vi "Reconnected.vi"(8 "error in (no error)":errorcluster, 11 "PolledDriver in":refnum<class "PolledDriver.lvclass">) -> (0 "error out":errorcluster, 3 "PolledDriver out":refnum<class "PolledDriver.lvclass">)   [LabVIEW 2013, in "PolledDriver.lvclass"]
doc: "Called when driver has sucesfully reconnected to host"
uses:
  PolledDriver.lvclass
  response.ctl
  driver_status.ctl
  Responder/BaseResponder/BaseResponder.lvclass
  PolledDriver.lvclass/PolledDriver.ctl
  BaseDriver/Read Responder.vi
  BaseDriver/Write Responder.vi
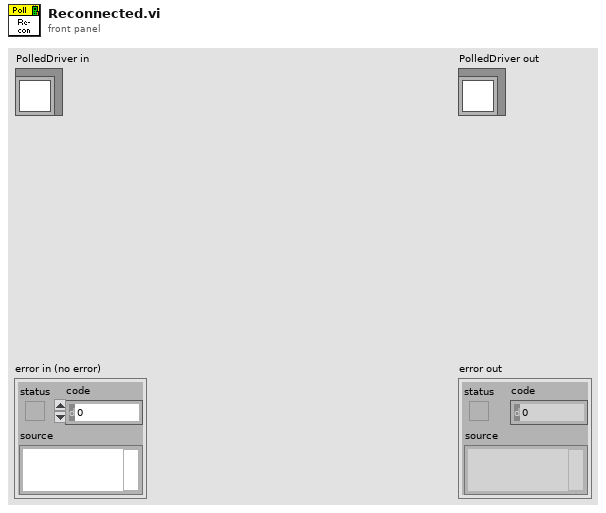
[diagram p1: front panel]
types:
  T1 = typedef "driver_status.ctl" = enum16{"Normal", "Startup", "Connection lost", "Reconnected", "Timeout", "Idle", "Busy"}
  T2 = typedef "response.ctl" = cluster{"driver status":T1, "Sender":string, "Type":i32, "Variant":variant}
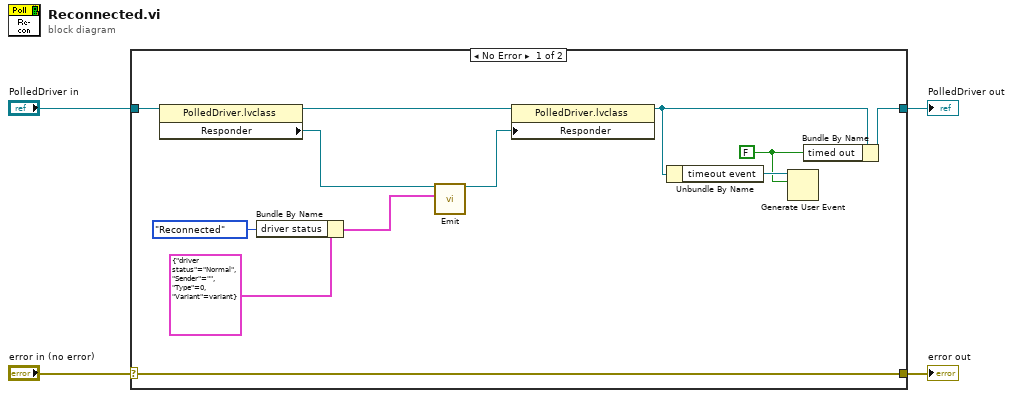
[diagram p0: block diagram]
diagram:
  n1 = case shown="No Error" "error in (no error)" {
    selector: "error in (no error)" -> [w16 w18]
    tunnel: [w16 w18] -> w3
    tunnel: [w11 w17] -> w1
    tunnel: "PolledDriver in" -> [w15 w17]
    frame No Error {
      w8 = FALSE ("timed out")
      n2 = property on="Property Node" class="PolledDriver.lvclass"(reference=w15) -> (reference out=w14:refnum<class "PolledDriver.lvclass">, "Responder"=w13:refnum<class "BaseResponder.lvclass">)  [unwired: 1 in, 1 out]
      n3 = Bundle By Name(cluster=T2 {"driver status"=enum."Normal", "Sender"="", "Type"=0, "Variant"=variant} ("response"), "driver status"=driver_status."Reconnected") -> (w5:T2)
      n4 = call-dynamic "Emit.vi"("response"=w5, "BaseResponder in"=w13) -> ("BaseResponder out"=w12:refnum<class "BaseResponder.lvclass">)  [unwired: 8 in, 1 out]
      n5 = property on="Property Node" class="PolledDriver.lvclass"(reference=w14, "Responder"=w12) -> (reference out=w9:refnum<class "PolledDriver.lvclass">)  [unwired: 1 in, 1 out]
      n6 = Unbundle By Name(w9) -> ("timeout event"=w10:refnum<user-event>)
      n7 = Generate User Event(user event=w10, event data cluster=w8) -> ()  [unwired: 2 in, 2 out]
      n8 = Bundle By Name(cluster=w9, "timed out"=w8) -> (w11:refnum<class "PolledDriver.lvclass">)
    }
    frame Error {
    }
  }
  "error out" <- w3
  "PolledDriver out" <- w1
